vi "GetSpectrum.vi"(0 "Acquire / Pause? External":refnum<vi>, 1 "% averaged (external)":refnum<vi>, 2 "Binned interferogram (external)":refnum<vi>, 5 "N delays":i32=30000, 7 "Acquisition cycle (external)":refnum<vi>, 9 "Delay calibration\n          factor":dbl=2.403, 11 "Subtract\ndelay (ps)":dbl=0.45, 12 "Acquisitions per interferogram":i32=2, 13 "Time per acquisition (s)":dbl=1.0, 14 "Sampling rate":dbl=250000.0, 15 "Extract envelope":bool=TRUE) -> (4 "Output spectrum":dbl[][](array[numeric]), 6 "Python error":errorcluster)   [LabVIEW 2021]
uses:
  Control_AcquireSpectrum.ctl
  <vilib>/Analysis/Matrix/Numeric/Conversions/Matrix To Array - RM.vi
  <vilib>/Analysis/Matrix/NI_Matrix.lvlib
panel:
  out "Refnum errors":errorcluster={"status"=TRUE, "code"=91, "source"="Property Node (arg 1) in GetSpectrum.vi->ScanDelay_DAQ_Fourier_test.vi\n<APPEND>\nProperty Name: <b>Value</b>"}
  out "Spectrum (amplitude)":cluster{dbl[], dbl[]}[](graph)
  out "Spectrum (phase)":cluster{dbl[], dbl[]}(graph)
  out "Interferogram (binned)":cluster{dbl, dbl}[](graph)
  in  "Acquire / pause?":bool=TRUE
  out "% averaged":dbl=100.0
  out "Acquisition cycle":dbl[][](graph)
  in  "Halt acquisition":bool
  out "Python module path":path=path "C:/Users/mnopl/Desktop/Software/LabVIEW/ScanDelay/scandelay.py"
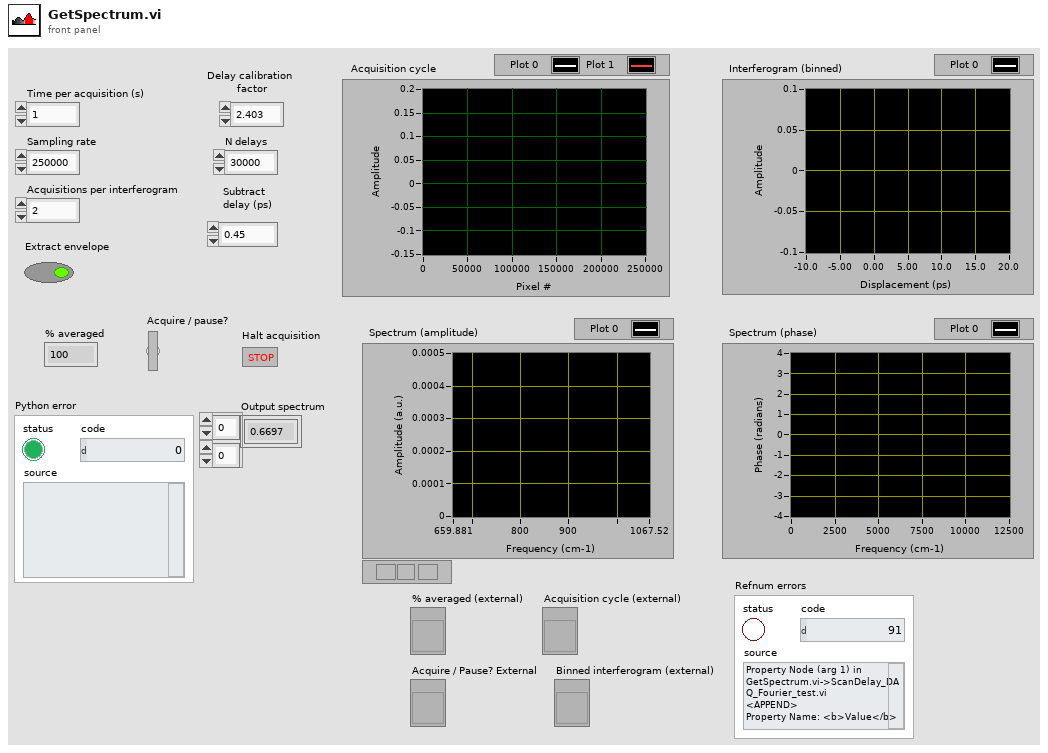
[diagram p1: front panel]
types:
  T1 = typedef "Control_AcquireSpectrum.ctl" = enum16{"Acquire Interferogram", "Bin Interferogram", "Compute Spectrum", "Done"}
  T2 = typedef "NI_Matrix.lvlib/RealMatrix.ctl" = dbl[][]
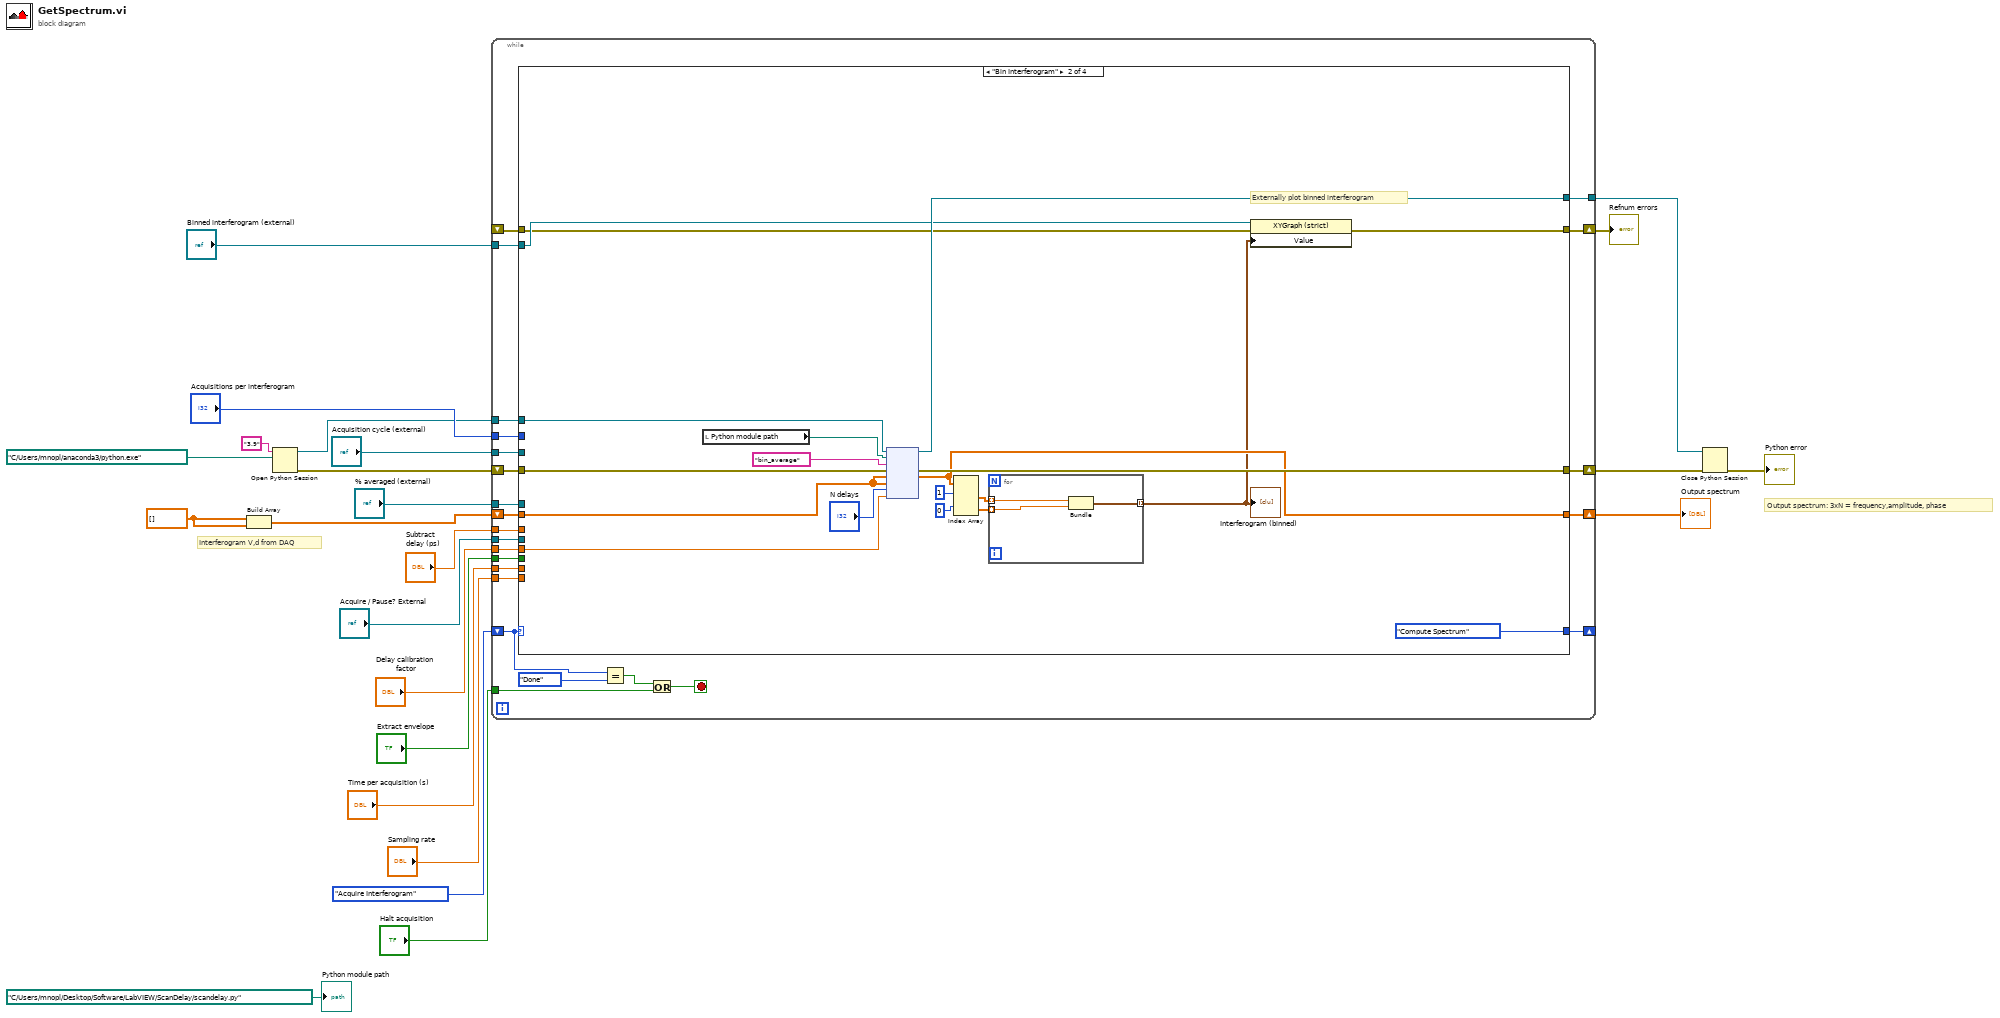
[diagram p0: block diagram]
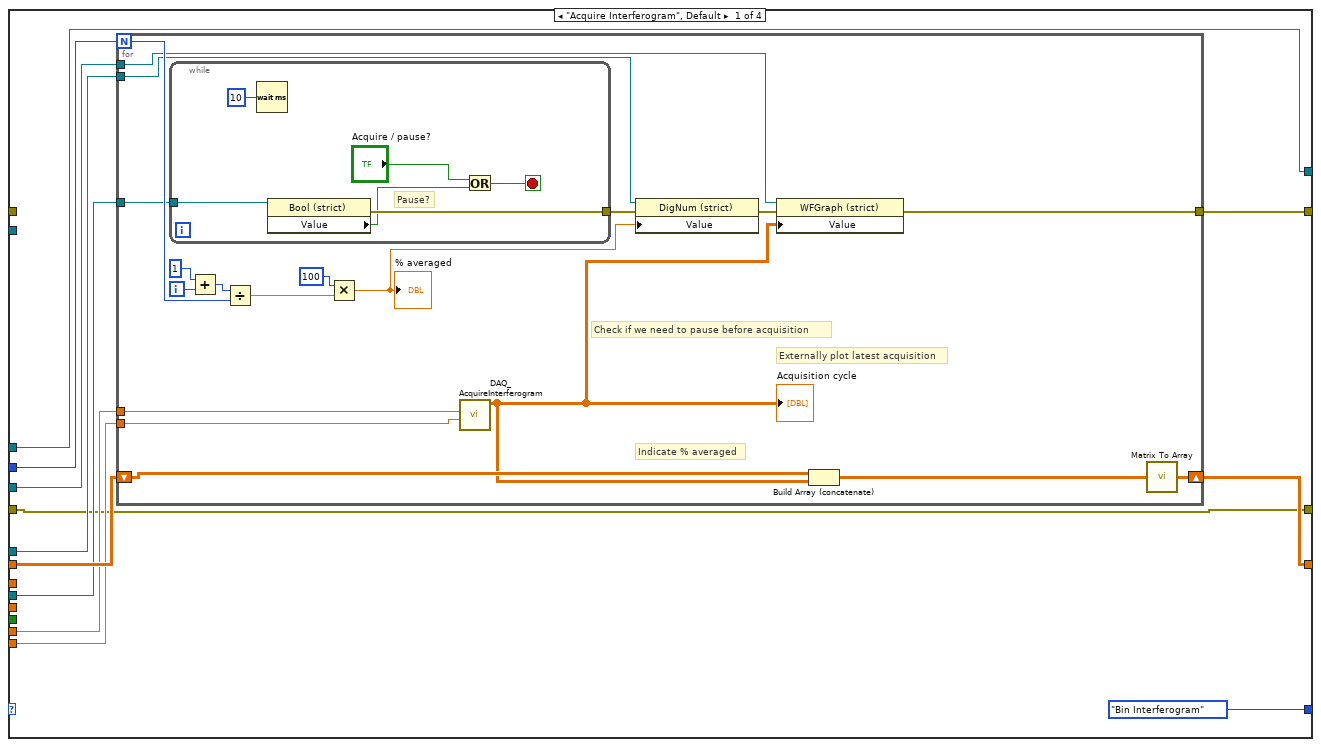
[diagram p2: hidden frame]
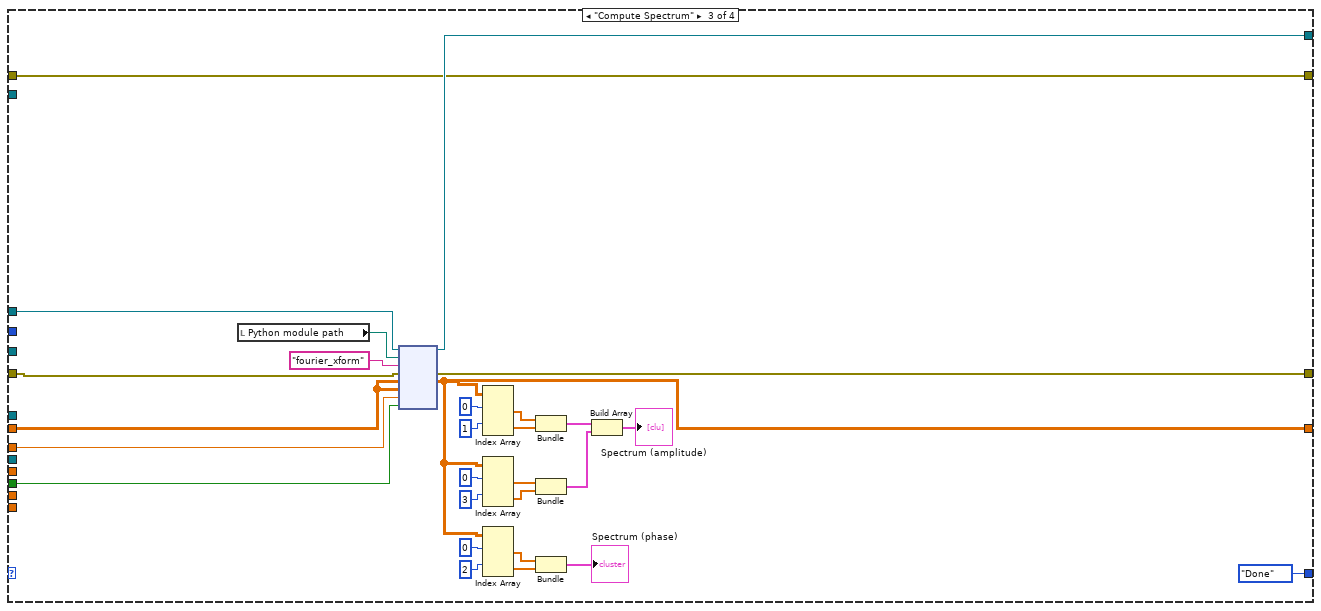
[diagram p3: hidden frame]
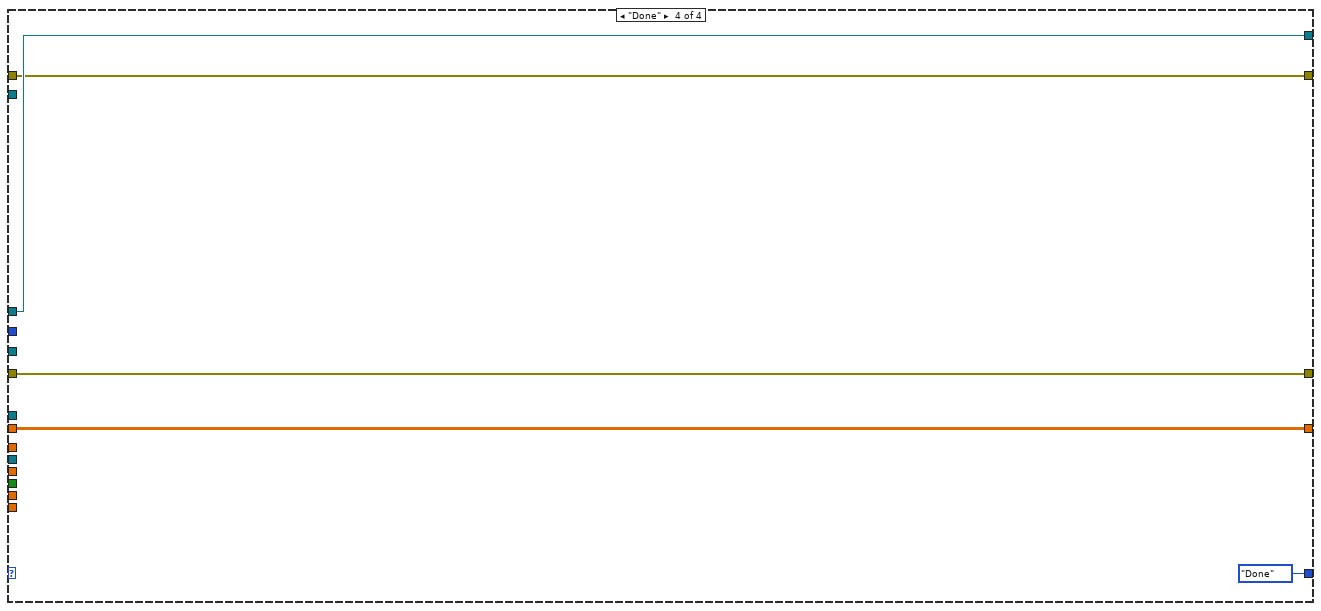
[diagram p4: hidden frame]
diagram:
  w7 = dbl[] []
  # "Output spectrum: 3xN = frequency,amplitude, phase"
  # "Interferogram V,d from DAQ"
  n1 = Build Array(w7, w7) -> (w6:dbl[][])
  n2 = Open Python Session(python version="3.9", python path=path "C:/Users/mnopl/anaconda3/python.exe") -> (session out=w16:refnum<k35>, error out=w17:errorcluster)  [unwired: 1 in]
  n3 = while {
    shift-right: [w48] -> w5
    shift-left: w6 -> [w47]
    tunnel: w16 -> [w46]
    tunnel: "Acquisition cycle (external)" -> [w44]
    tunnel: "Sampling rate" -> [w43]
    tunnel: "Time per acquisition (s)" -> [w42]
    tunnel: "Delay calibration\n          factor" -> [w41]
    tunnel: "% averaged (external)" -> [w40]
    tunnel: "Acquire / Pause? External" -> [w39]
    tunnel: "Acquisitions per interferogram" -> [w38]
    shift-right: [w37] -> _
    shift-left: Control_AcquireSpectrum."Acquire Interferogram" -> [w35]
    tunnel: "Subtract\ndelay (ps)" -> [w36]
    tunnel: "Halt acquisition" -> [w33]
    tunnel: [w30] -> w9
    shift-right: [w29] -> w4
    shift-left: w17 -> [w45]
    tunnel: "Extract envelope" -> [w28]
    shift-right: [w27] -> w2
    shift-left: _ -> [w26]
    tunnel: "Binned interferogram (external)" -> [w25]
    stop <- w31 stop-if-true
    n4 = case shown="\"Bin Interferogram\"" w35 {
      tunnel: [w60 w89 w113 w140] -> w48
      tunnel: w47 -> [w59 w102 w134 w140]
      tunnel: w46 -> [w51 w101 w133 w138]
      tunnel: w45 -> [w50 w100 w130 w139]
      tunnel: w44 -> [w58 _ _ _]
      tunnel: w43 -> [w57 _ _ _]
      tunnel: w42 -> [w56 _ _ _]
      tunnel: w41 -> [_ w99 _ _]
      tunnel: w40 -> [w55 _ _ _]
      tunnel: w39 -> [w54 _ _ _]
      tunnel: w38 -> [w53 _ _ _]
      tunnel: [w51 w98 w132 w138] -> w30
      tunnel: [Control_AcquireSpectrum."Bin Interferogram" Control_AcquireSpectrum."Compute Spectrum" Control_AcquireSpectrum."Done" Control_AcquireSpectrum."Done"] -> w37
      tunnel: w36 -> [_ _ w129 _]
      tunnel: [w50 w93 w119 w139] -> w29
      tunnel: w28 -> [_ _ w118 _]
      tunnel: [w49 w90 w108 w136] -> w27
      tunnel: w26 -> [_ w91 w108 w136]
      tunnel: w25 -> [_ w92 _ _]
      frame "Acquire Interferogram", Default {
        n5 = for {
          N: w53 -> [w71]
          shift-right: [w78] -> w60
          shift-left: w59 -> [w77]
          tunnel: w58 -> [w64]
          tunnel: w57 -> [w70]
          tunnel: w56 -> [w69]
          tunnel: w55 -> [w68]
          tunnel: w54 -> [w67]
          tunnel: [w61] -> w49
          i -> [w72]
          # "Externally plot latest acquisition"
          # "Indicate % averaged"
          # "Check if we need to pause before acquisition"
          n6 = while {
            tunnel: w67 -> [w84]
            tunnel: [w82] -> w62
            stop <- w83 stop-if-true
            # "Pause?"
            n7 = Wait (ms)(milliseconds to wait=10) -> ()  [unwired: 1 out]
            n8 = property on="Property Node" class="Bool (strict)"(reference=w84) -> (error out=w82:errorcluster, "Value"=w81:bool)  [unwired: 1 in, 1 out]
            n9 = Or(x="Acquire / pause?", y=w81) -> (x .or. y?=w83:bool)
          }
          n10 = Add(x=1, y=w72) -> (x+y=w75:i32)
          n11 = Divide(x=w75, y=w71) -> (x/y=w76:dbl)
          n12 = Multiply(x=100, y=w76) -> (x*y=w66:dbl)
          "% averaged" <- w66
          n13 = call "DAQ_AcquireInterferogram.vi"("Sampling rate"=w70, "Time per acquisiton (s)"=w69) -> ("Output V-d array"=w65:dbl[][])  [unwired: 9 in]
          "Acquisition cycle" <- w65
          n14 = property on="Property Node" class="DigNum (strict)"(reference=w68, error in=w62, "Value"=w66) -> (error out=w63:errorcluster)  [unwired: 1 out]
          n15 = property on="Property Node" class="WFGraph (strict)"(reference=w64, error in=w63, "Value"=w65) -> (error out=w61:errorcluster)  [unwired: 1 out]
          n16 = Build Array (concatenate)(w77, w65) -> (w79:T2)
          n17 = call-poly <vilib>:"Matrix To Array.vi"("Real Matrix"=w79) -> ("Real 2D Array"=w78:dbl[][])
        }
      }
      frame "Bin Interferogram" {
        # "Externally plot binned interferogram"
        n18 = local read "Python module path"() -> (w97:path)
        n19 = node(w101, w97, "bin_average", w100, w102, w102, "N delays", w99) -> (w98:refnum<k35>, w93:errorcluster, w89:dbl[][])  [unwired: 3 in, 2 out]
        n20 = Index Array(array=w89, index (row) #1=1, index (row) #2=0) -> (element #1=w87:dbl[], element #2=w88:dbl[])  [unwired: 2 in]
        n21 = for {
          tunnel: w88 -> [w106] mode=indexing
          tunnel: w87 -> [w107] mode=indexing
          tunnel: [w105] -> w86 mode=indexing
          n22 = Bundle(w107, w106) -> (w105:cluster{dbl, dbl})  [unwired: 1 in]
        }
        "Interferogram (binned)" <- w86
        n23 = property on="Property Node" class="XYGraph (strict)"(reference=w92, error in=w91, "Value"=w86) -> (error out=w90:errorcluster)  [unwired: 1 out]
      }
      frame "Compute Spectrum" {
        n24 = local read "Python module path"() -> (w131:path)
        n25 = node(w133, w131, "fourier_xform", w130, w134, w134, w129, w118) -> (w132:refnum<k35>, w119:errorcluster, w113:dbl[][])  [unwired: 3 in, 2 out]
        n26 = Index Array(array=w113, index (row) #1=0, index (row) #2=1) -> (element #1=w125:dbl[], element #2=w124:dbl[])  [unwired: 2 in]
        n27 = Index Array(array=w113, index (row) #1=0, index (row) #2=3) -> (element #1=w120:dbl[], element #2=w121:dbl[])  [unwired: 2 in]
        n28 = Index Array(array=w113, index (row) #1=0, index (row) #2=2) -> (element #1=w114:dbl[], element #2=w115:dbl[])  [unwired: 2 in]
        n29 = Bundle(w125, w124) -> (w111:cluster{dbl[], dbl[]})  [unwired: 1 in]
        n30 = Bundle(w120, w121) -> (w110:cluster{dbl[], dbl[]})  [unwired: 1 in]
        n31 = Bundle(w114, w115) -> (→"Spectrum (phase)":cluster{dbl[], dbl[]})  [unwired: 1 in]
        n32 = Build Array(w111, w110) -> (→"Spectrum (amplitude)":cluster{dbl[], dbl[]}[])
      }
      frame "Done" {
      }
    }
    n33 = Equal?(x=w35, y=Control_AcquireSpectrum."Done") -> (x = y?=w32:bool)
    n34 = Or(x=w32, y=w33) -> (x .or. y?=w31:bool)
  }
  "Output spectrum" <- w5
  "Refnum errors" <- w2
  n35 = Close Python Session(session in=w9, error in=w4) -> (11:→"Python error":errorcluster)
  "Python module path" <- path "C:/Users/mnopl/Desktop/Software/LabVIEW/ScanDelay/scandelay.py"
